vi "SetDriveSpeedDmd.vi"(8 "LeftSpeedInput":dbl, 11 "RightSpeedInput":dbl) -> ()   [LabVIEW 2020]
uses:
  DriveGlobals.vi
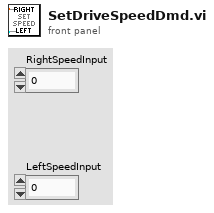
[diagram p1: front panel]
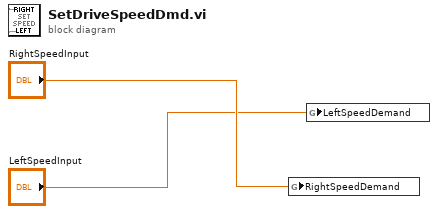
[diagram p0: block diagram]
diagram:
  n1 = global write "DriveGlobals.vi" "RightSpeedDemand"("RightSpeedInput") -> ()
  n2 = global write "DriveGlobals.vi" "LeftSpeedDemand"("LeftSpeedInput") -> ()
